vi "Eth Status Read Start.vi"(7 "Status Reference":T1, 8 "error in (no error)":errorcluster, 11 "N":i32) -> (0 "error out":errorcluster, 1 "Start":bool)   [LabVIEW 2019, in "Eth Status.lvlib"]
uses:
  Eth Status.lvlib
  Ctl/ICPCON Status.ctl
  MB_TCP2/MB_TCP_State.ctl
  MB_TCP2/MB_TCP.lvclass
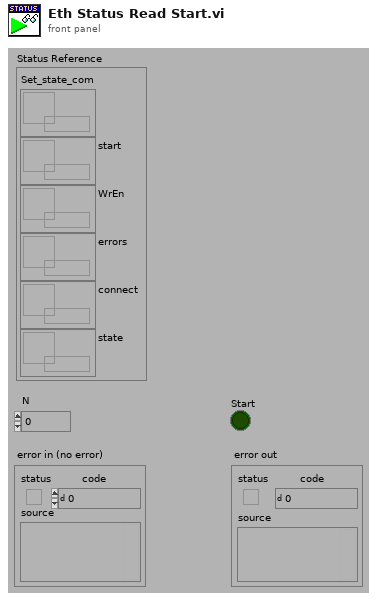
[diagram p1: front panel]
types:
  T1 = typedef "Eth Status.lvlib/ICPCON Status.ctl" = cluster{"Set_state_com":refnum<data-value>, "start":refnum<data-value>, "WrEn":refnum<data-value>, "errors":refnum<data-value>, "connect":refnum<data-value>, "state":refnum<data-value>}
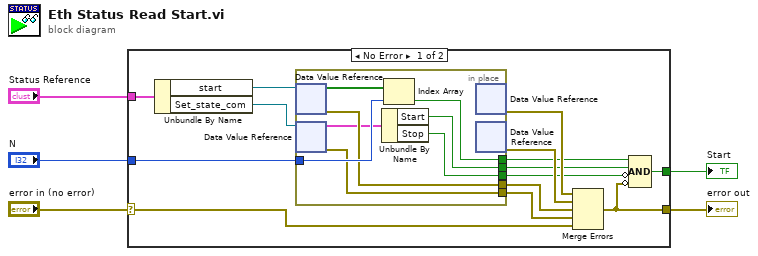
[diagram p0: block diagram]
diagram:
  n1 = case shown="No Error" "error in (no error)" {
    selector: "error in (no error)" -> [w11 w28]
    tunnel: [w9 w28] -> w5
    tunnel: [w10 _] -> w2
    tunnel: "N" -> [w19 _]
    tunnel: "Status Reference" -> [w18 _]
    frame No Error {
      n2 = Unbundle By Name(w18) -> ("start"=w16:refnum<data-value>, "Set_state_com"=w15:refnum<data-value>)
      n3 = in-place {
        in-place-border: w19 -> [w27]
        in-place-border: [w25] -> w13
        in-place-border: [w24] -> w12
        in-place-border: [w21] -> w7
        in-place-border: [w23] -> w8
        in-place-border: [w20] -> w6
        n4 = in-place-dvr #1(w16) -> (w26:bool[], w25:errorcluster)
        n5 = in-place-dvr #2(w15) -> (w22:cluster{"Start":bool, "WrEn":bool, "Stop":bool}, w24:errorcluster)
        n6 = Unbundle By Name(w22) -> ("Start"=w21:bool, "Stop"=w20:bool)
        n7 = Index Array(array=w26, index=w27) -> (element=w23:bool)
        n8 = in-place-dvr #1() -> (w17:errorcluster)  [unwired: 1 in, 1 out]
        n9 = in-place-dvr #2() -> (w14:errorcluster)  [unwired: 1 in, 1 out]
      }
      n10 = Merge Errors(w17, w14, w13, w12, w11) -> (w9:errorcluster)
      n11 = Compound Arithmetic op=AND(w8, w7, invert w6, invert w9) -> (w10:bool)
    }
    frame Error {
    }
  }
  "error out" <- w5
  "Start" <- w2
